vi "Command Robot.vi"(11 "all rows":dbl[][](array[numeric]) format="%_6g") -> ()   [LabVIEW 2020]
panel:
  out "X-DriveAuto":dbl
  out "Y-DriveAuto":dbl
  out "Control Panel":bool
  out "Climb":bool
  out "Intake":bool
  out "Shooter":bool
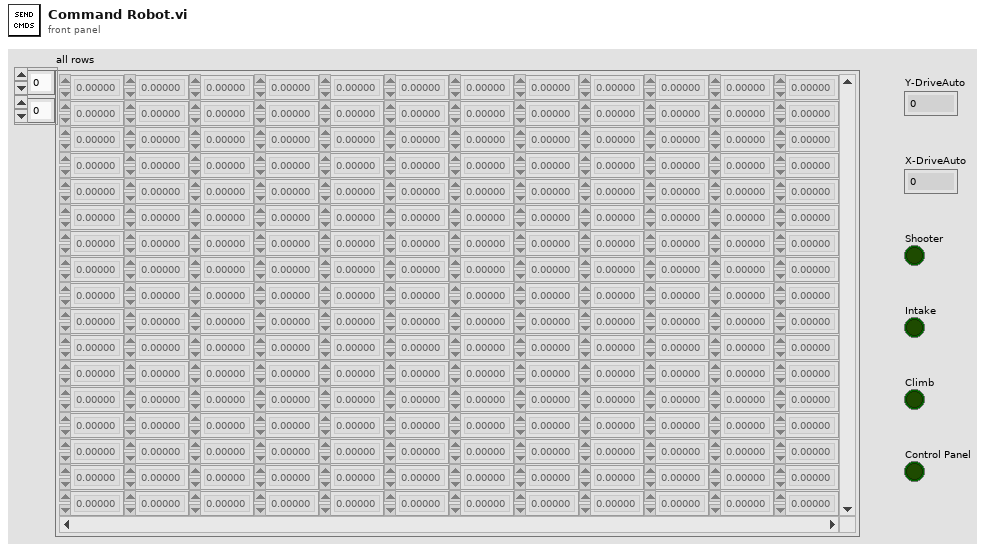
[diagram p1: front panel]
types:
  T1 = typedef "Command Status Info.ctl" = cluster{"Name":string, "Status":T2, "notifier out":T3}
  T2 = typedef "Completion Status.ctl" = enum16{"Successful", "Aborted", "Incomplete"}
  T3 = typedef "Completion Notifier.ctl" = refnum<notifier>
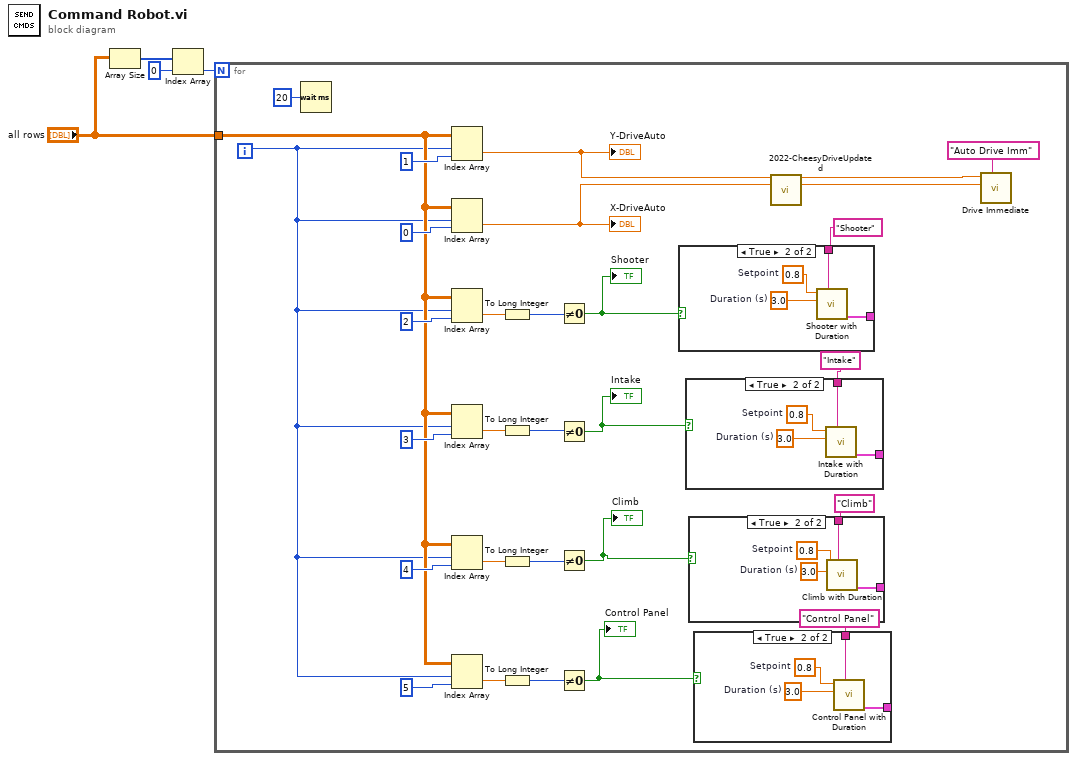
[diagram p0: block diagram]
diagram:
  n1 = Array Size(array="all rows") -> (size(s)=w2:i32[])
  n2 = Index Array(array=w2, index=0) -> (element=w1:i32)
  n3 = for {
    N: w1 -> [_]
    tunnel: "all rows" -> [w24]
    i -> [w23]
    n4 = Wait (ms)(milliseconds to wait=u32 20) -> ()  [unwired: 1 out]
    n5 = Index Array(array=w24, index (row)=w23, index (col)=1 ("disabled index (col)")) -> (element=w14:dbl)
    "Y-DriveAuto" <- w14
    n6 = Index Array(array=w24, index (row)=w23, index (col)=0 ("disabled index (col)")) -> (element=w13:dbl)
    "X-DriveAuto" <- w13
    n7 = Index Array(array=w24, index (row)=w23, index (col)=2 ("disabled index (col)")) -> (element=w28:dbl)
    n8 = Index Array(array=w24, index (row)=w23, index (col)=3 ("disabled index (col)")) -> (element=w30:dbl)
    n9 = Index Array(array=w24, index (row)=w23, index (col)=4 ("disabled index (col)")) -> (element=w32:dbl)
    n10 = Index Array(array=w24, index (row)=w23, index (col)=5 ("disabled index (col)")) -> (element=w34:dbl)
    n11 = To Long Integer(number=w28) -> (32bit integer=w22:i32)
    n12 = To Long Integer(number=w30) -> (32bit integer=w21:i32)
    n13 = To Long Integer(number=w32) -> (32bit integer=w20:i32)
    n14 = To Long Integer(number=w34) -> (32bit integer=w19:i32)
    n15 = Not Equal To 0?(x=w22) -> (x != 0?=w8:bool)
    "Shooter" <- w8
    n16 = Not Equal To 0?(x=w21) -> (x != 0?=w7:bool)
    "Intake" <- w7
    n17 = Not Equal To 0?(x=w20) -> (x != 0?=w6:bool)
    "Climb" <- w6
    n18 = Not Equal To 0?(x=w19) -> (x != 0?=w5:bool)
    "Control Panel" <- w5
    n19 = case shown="True" w8 {
      tunnel: [_ w50] -> _
      tunnel: "Shooter" ("Description") -> [_ w49]
      frame False {
      }
      frame True {
        w47 = 3.0  # Duration (s)
        w48 = 0.8  # Setpoint
        n20 = call "Shooter with Duration.vi"("Description"=w49, "Duration (s)"=w47, "Setpoint"=w48) -> ("Command Info Out"=w50:T1)  [unwired: 8 in]
      }
    }
    n21 = case shown="True" w7 {
      tunnel: [_ w46] -> _
      tunnel: "Intake" ("Description") -> [_ w45]
      frame False {
      }
      frame True {
        w43 = 3.0  # Duration (s)
        w44 = 0.8  # Setpoint
        n22 = call "Intake with Duration.vi"("Description"=w45, "Duration (s)"=w43, "Setpoint"=w44) -> ("Command Info Out"=w46:T1)  [unwired: 8 in]
      }
    }
    n23 = case shown="True" w6 {
      tunnel: [_ w42] -> _
      tunnel: "Climb" ("Description") -> [_ w41]
      frame False {
      }
      frame True {
        w39 = 0.8  # Setpoint
        w40 = 3.0  # Duration (s)
        n24 = call "Climb with Duration.vi"("Description"=w41, "Duration (s)"=w40, "Setpoint"=w39) -> ("Command Info Out"=w42:T1)  [unwired: 8 in]
      }
    }
    n25 = case shown="True" w5 {
      tunnel: [_ w38] -> _
      tunnel: "Control Panel" ("Description") -> [_ w37]
      frame False {
      }
      frame True {
        w35 = 3.0  # Duration (s)
        w36 = 0.8  # Setpoint
        n26 = call "Control Panel with Duration.vi"("Description"=w37, "Duration (s)"=w35, "Setpoint"=w36) -> ("Command Info Out"=w38:T1)  [unwired: 8 in]
      }
    }
    n27 = call "2022-CheesyDriveUpdated.vi"("Throttle"=w14, "Wheel"=w13) -> ("Left PWM"=w16:dbl, "Right PWM"=w17:dbl)  [unwired: 11 in, 1 out]
    n28 = call "Drive Immediate.vi"("Description"="Auto Drive Imm", "Right Setpoint"=w17, "Left Setpoint"=w16) -> ()  [unwired: 8 in, 1 out]
  }
